vi "CreateGraphMenu_OnGraphYaxle.vi"(11 "菜单输入":refnum<k9>) -> ()   [LabVIEW 2015]
uses:
  GlobalVariables.vi
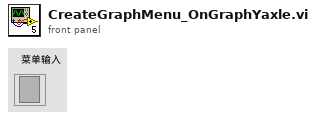
[diagram p1: front panel]
types:
  T1 = cluster{"MenuNames":string[], "MenuTags":string[]}
  T2 = cluster{"Ylimits":cluster{"Upbound":dbl, "Downbound":dbl}, "ParentScaleID":i32, "LabelTitle":string}
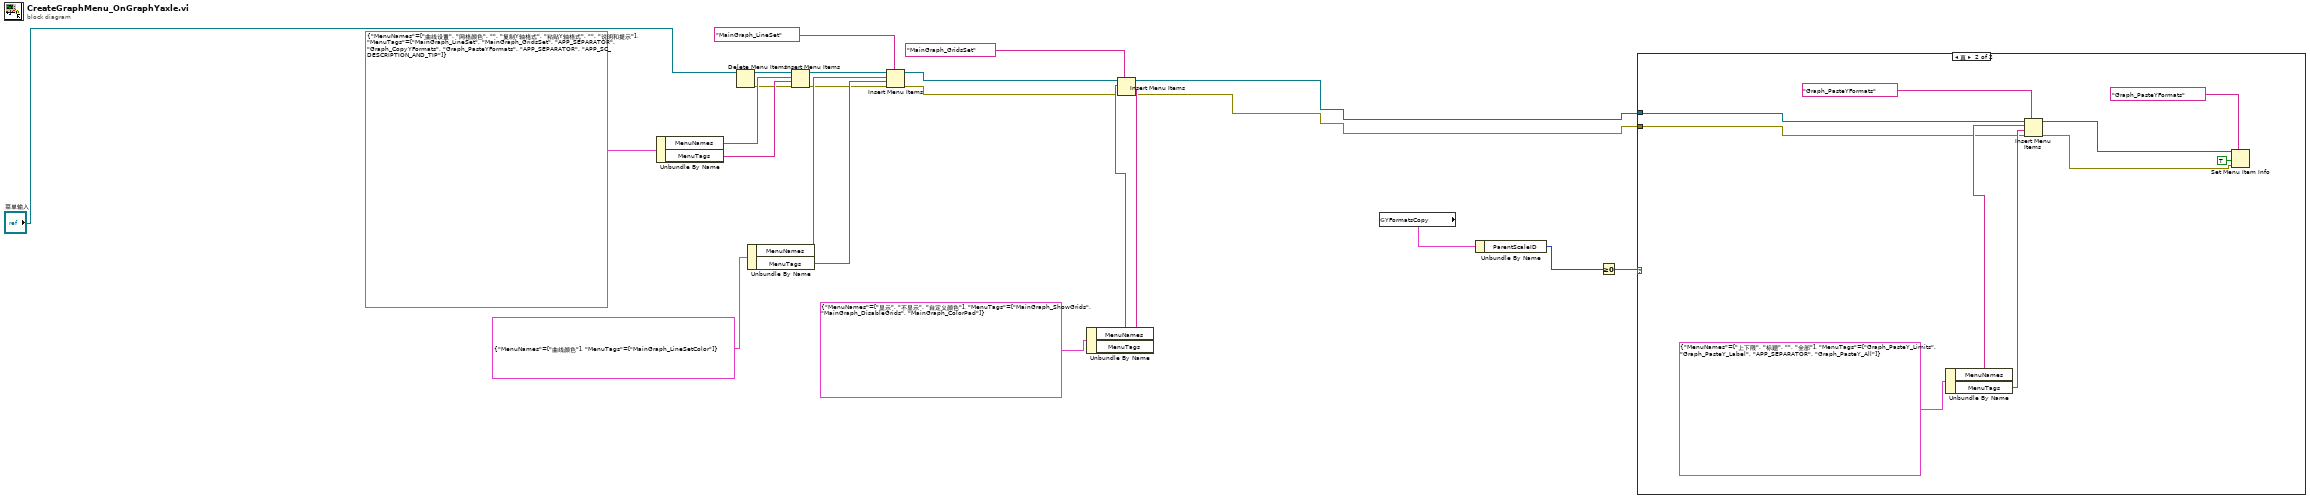
[diagram p0: block diagram]
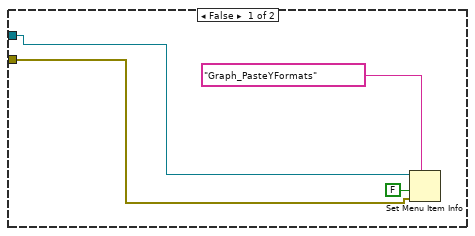
[diagram p2: hidden frame]
diagram:
  n1 = Unbundle By Name(T1 {"MenuNames"=["曲线设置", "网格颜色", "", "复制Y轴格式", "粘贴Y轴格式", "", "说明和提示"], "MenuTags"=["MainGraph_LineSet", "MainGraph_GridsSet", "APP_SEPARATOR", "Graph_CopyYFormats", "Graph_PasteYFormats", "APP_SEPARATOR", "APP_SC_DESCRIPTION_AND_TIP"]}) -> ("MenuNames"=w15:string[], "MenuTags"=w16:string[])
  n2 = Delete Menu Items(9:"菜单输入") -> (0:w6:errorcluster, 3:w9:refnum<k9>)  [unwired: 3 in]
  n3 = Unbundle By Name(T1 {"MenuNames"=["曲线颜色"], "MenuTags"=["MainGraph_LineSetColor"]}) -> ("MenuNames"=w19:string[], "MenuTags"=w18:string[])
  n4 = Insert Menu Items(6:w6, 7:w16, 8:w15, 9:w9) -> (0:w8:errorcluster, 3:w13:refnum<k9>)  [unwired: 2 in, 1 out]
  n5 = Insert Menu Items(5:"MainGraph_LineSet" ("L10n_menu tag"), 6:w8, 7:w18, 8:w19, 9:w13) -> (0:w7:errorcluster, 3:w12:refnum<k9>)  [unwired: 1 in, 1 out]
  n6 = Unbundle By Name(T1 {"MenuNames"=["显示", "不显示", "自定义颜色"], "MenuTags"=["MainGraph_ShowGrids", "MainGraph_DisableGrids", "MainGraph_ColorPad"]}) -> ("MenuNames"=w21:string[], "MenuTags"=w22:string[])
  n7 = Insert Menu Items(5:"MainGraph_GridsSet" ("L10n_menu tag"), 6:w7, 7:w22, 8:w21, 9:w12) -> (0:w1:errorcluster, 3:w2:refnum<k9>)  [unwired: 1 in, 1 out]
  n8 = global read "GlobalVariables.vi" "YFormatsCopy"() -> (w5:T2)
  n9 = Unbundle By Name(w5) -> ("ParentScaleID"=w4:i32)
  n10 = Greater Or Equal To 0?(x=w4) -> (x >= 0?=w3:bool)
  n11 = case shown="真" w3 {
    tunnel: w1 -> [w24 w33]
    tunnel: w2 -> [w27 w32]
    frame False {
      n12 = Set Menu Item Info(7:"Graph_PasteYFormats" ("L10n_menu tag"), 8:w24, 9:FALSE ("已启用"), 11:w27) -> ()  [unwired: 3 in, 2 out]
    }
    frame True {
      n13 = Unbundle By Name(T1 {"MenuNames"=["上下限", "标题", "", "全部"], "MenuTags"=["Graph_PasteY_Limits", "Graph_PasteY_Label", "APP_SEPARATOR", "Graph_PasteY_All"]}) -> ("MenuNames"=w35:string[], "MenuTags"=w34:string[])
      n14 = Insert Menu Items(5:"Graph_PasteYFormats" ("L10n_menu tag"), 6:w33, 7:w34, 8:w35, 9:w32) -> (0:w28:errorcluster, 3:w29:refnum<k9>)  [unwired: 1 in, 1 out]
      n15 = Set Menu Item Info(7:"Graph_PasteYFormats" ("L10n_menu tag"), 8:w28, 9:TRUE ("已启用"), 11:w29) -> ()  [unwired: 3 in, 2 out]
    }
  }
